vi "get_configuration_paths.vi"(8 "error in (no error)":errorcluster, 10 "file name (without ending)":string, 11 "GenericComponent in":refnum<class "GenericComponent.lvclass">) -> (0 "error out":errorcluster, 1 "configuration file path":path, 2 "configuration directory for a specific component":path, 3 "GenericComponent out":refnum<class "GenericComponent.lvclass">, 4 "main configuration file path":path, 5 "configuration directory for a specific user":path, 6 "main configuration directory":path, 7 "configuration base directory":path)   [LabVIEW 2011, in "GenericComponent.lvclass"]
uses:
  GenericComponent.lvclass
  xcontrols/XUserDropdown/XUserDropdown/XUserDropdown.xctl
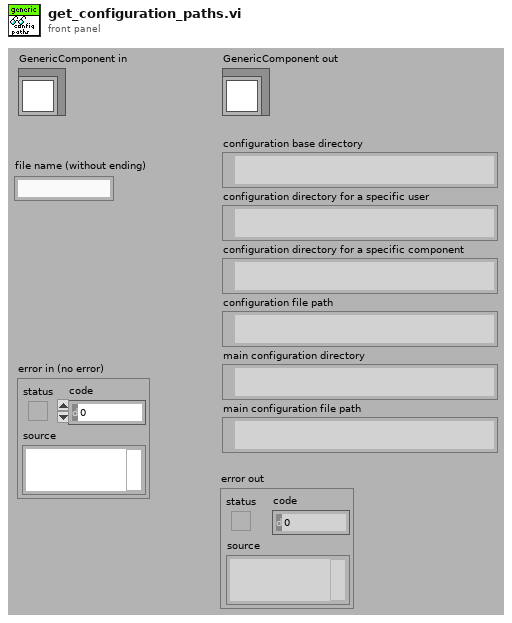
[diagram p1: front panel]
types:
  T1 = typedef "plugin_specification.ctl" = cluster{"class path":string, "configuration":string, "label":string, "settings name":string}
  T2 = typedef "configuration_paths_cluster.ctl" = cluster{"base folder":path, "base folder for user":path, "component folder":path, "component file path":path, "main folder":path, "main file":path}
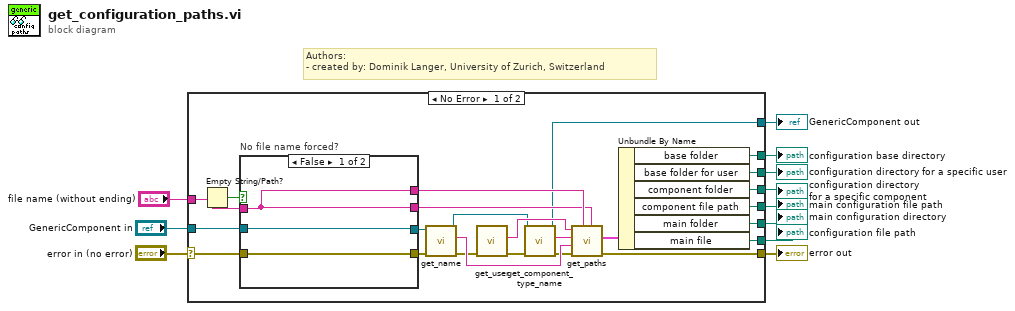
[diagram p0: block diagram]
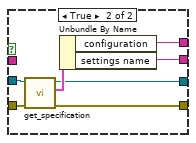
[diagram p2: hidden frame]
diagram:
  # "Authors: \n- created by: Dominik Langer, University of Zurich, Switzerland"
  n1 = case shown="No Error" "error in (no error)" {
    selector: "error in (no error)" -> [w24 w47]
    tunnel: [w21 w47] -> w10
    tunnel: [w22 w46] -> w8
    tunnel: "GenericComponent in" -> [w23 w46]
    tunnel: [w19 _] -> w7
    tunnel: [w18 _] -> w5
    tunnel: [w17 _] -> w6
    tunnel: [w16 _] -> w4
    tunnel: [w15 _] -> w3
    tunnel: [w14 _] -> w2
    tunnel: "file name (without ending)" -> [w13 _]
    frame No Error {
      n2 = Empty String/Path?(string/path=w13) -> (empty?=w25:bool)
      n3 = case "No file name forced?" shown="False" w25 {
        tunnel: w24 -> [w37 w45]
        tunnel: [w37 w43] -> w33
        tunnel: w23 -> [w38 w44]
        tunnel: [w36 w40] -> w35
        tunnel: [w38 w39] -> w32
        tunnel: w13 -> [w36 _]
        tunnel: [w36 w41] -> w34
        frame False {
        }
        frame True {
          n4 = call-dynamic "get_specification.vi"("error in (no error)"=w45, "GenericPlugin in"=w44) -> ("error out"=w43:errorcluster, "component specification"=w42:T1, "GenericPlugin out"=w39:refnum<class "GenericComponent.lvclass">)  [unwired: 6 in, 1 out]
          n5 = Unbundle By Name(w42) -> ("configuration"=w40:string, "settings name"=w41:string)
        }
      }
      n6 = call-dynamic "get_name.vi"("error in (no error)"=w33, "GenericPlugin in"=w32) -> ("error out"=w30:errorcluster, "component name"=w31:string, "GenericPlugin out"=w12:refnum<class "GenericComponent.lvclass">)  [unwired: 7 in]
      n7 = call "get_user.vi"("error in (no error)"=w30) -> ("error out"=w29:errorcluster, "username out"=w28:string)  [unwired: 9 in]
      n8 = call-dynamic "get_component_type_name.vi"("error in (no error)"=w29, "GenericPlugin in"=w12) -> ("error out"=w26:errorcluster, "component type"=w27:string, "GenericPlugin out"=w22:refnum<class "GenericComponent.lvclass">)  [unwired: 7 in]
      n9 = call "get_paths.vi"("settings file name (without ending)"=w34, "configuration file name (without ending)"=w35, "error in (no error)"=w26, "component name"=w31, "component type"=w27, "user"=w28) -> ("error out"=w21:errorcluster, "configuration paths"=w20:T2)  [unwired: 2 in, 2 out]
      n10 = Unbundle By Name(w20) -> ("base folder"=w19:path, "base folder for user"=w18:path, "component folder"=w17:path, "component file path"=w16:path, "main folder"=w15:path, "main file"=w14:path)
    }
    frame Error {
    }
  }
  "error out" <- w10
  "GenericComponent out" <- w8
  "configuration base directory" <- w7
  "configuration directory for a specific component" <- w6
  "configuration file path" <- w4
  "main configuration directory" <- w3
  "main configuration file path" <- w2
  "configuration directory for a specific user" <- w5
